vi "LTE Configure ModAcc.vi"(0 "RFmx Handle In":refnum<k21>, 1 "Selector String":string, 5 "RFmx LTE ModAcc Configuration":T1={"Synchronization Mode"=1, "Measurement Offset (slots)"=0, "Measurement Length (slots)"=1, "EVM Unit"=0, "Averaging Enabled"=0, "Averaging Count"=10} {"Averaging Enabled" items=["Percentage", "dB"]; "EVM Unit" items=["Percentage", "dB"]; "Synchronization Mode" items=["Frame", "Slot", "Marker"]}, 11 "error in (no error)":errorcluster) -> (4 "RFmx Handle Out":refnum<k21>, 15 "error out":errorcluster)   [LabVIEW 2016, in "RFmxLTE.lvlib"]
uses:
  RFmxLTE.lvlib
  Typedefs/LTE ModAcc Configuration.ctl
  <resource>/objmgr/RFmxLTE.rc
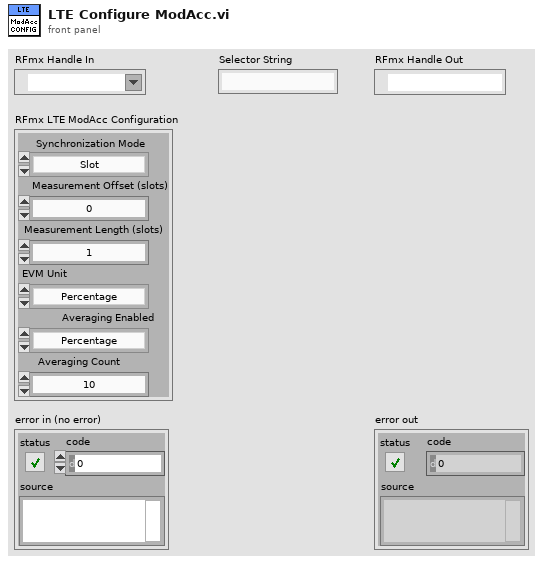
[diagram p1: front panel]
types:
  T1 = typedef "RFmxLTE.lvlib/LTE ModAcc Configuration.ctl" = cluster{"Synchronization Mode":i32, "Measurement Offset (slots)":i32, "Measurement Length (slots)":i32, "EVM Unit":i32, "Averaging Enabled":i32, "Averaging Count":i32}
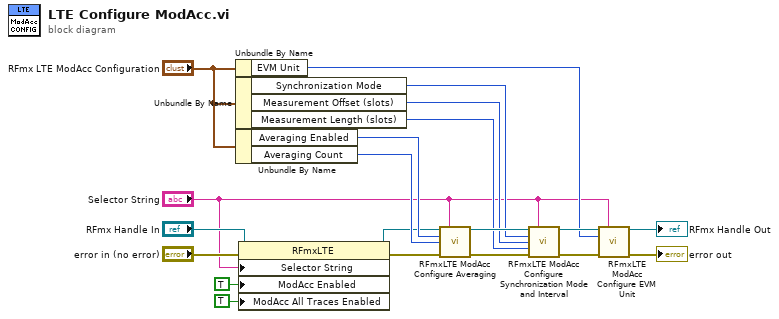
[diagram p0: block diagram]
diagram:
  n1 = Unbundle By Name("RFmx LTE ModAcc Configuration") -> ("EVM Unit"=w11:i32)
  n2 = Unbundle By Name("RFmx LTE ModAcc Configuration") -> ("Synchronization Mode"=w14:i32, "Measurement Offset (slots)"=w13:i32, "Measurement Length (slots)"=w12:i32)
  n3 = Unbundle By Name("RFmx LTE ModAcc Configuration") -> ("Averaging Enabled"=w10:i32, "Averaging Count"=w9:i32)
  n4 = property class="RFmxLTE"(reference="RFmx Handle In", error in="error in (no error)", "Selector String"="Selector String", "ModAcc Enabled"=TRUE, "ModAcc All Traces Enabled"=TRUE) -> (reference out=w7:refnum<k21>, error out=w8:errorcluster)
  n5 = call <vilib>:"RFmxLTE ModAcc Configure Averaging.vi"("Instrument Handle In"=w7, "Selector String"="Selector String", "Averaging Enabled"=w10, "Averaging Count"=w9, "error in (no error)"=w8) -> ("Instrument Handle Out"=w20:refnum<k21>, "error out"=w19:errorcluster)  [unwired: 9 in]
  n6 = call <vilib>:"RFmxLTE ModAcc Configure Synchronization Mode and Interval.vi"("Instrument Handle In"=w20, "Selector String"="Selector String", "Synchronization Mode"=w14, "Measurement Offset (slots)"=w13, "Measurement Length (slots)"=w12, "error in (no error)"=w19) -> ("Instrument Handle Out"=w18:refnum<k21>, "error out"=w17:errorcluster)  [unwired: 8 in]
  n7 = call <vilib>:"RFmxLTE ModAcc Configure EVM Unit.vi"("Instrument Handle In"=w18, "Selector String"="Selector String", "EVM Unit"=w11, "error in (no error)"=w17) -> ("Instrument Handle Out"=→"RFmx Handle Out":refnum<k21>, "error out"=→"error out":errorcluster)  [unwired: 10 in]
